vi "Authentication.vi"(2 "password":string, 3 "login":string, 4 "Server Data":string[][](array[string])) -> (0 "Index":i32, 1 "IsValid?":bool)   [LabVIEW 2016]
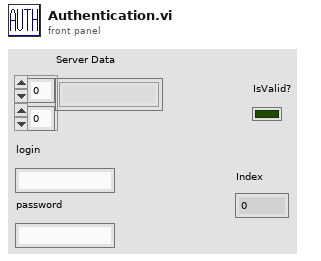
[diagram p1: front panel]
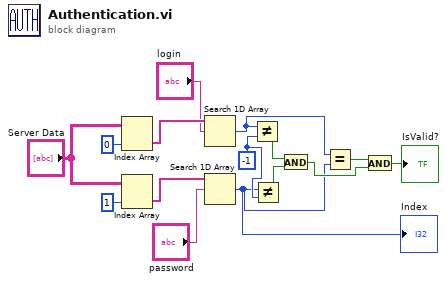
[diagram p0: block diagram]
diagram:
  w8 = -1
  n1 = Index Array(array="Server Data", index (col)=0) -> (element=w12:string[])  [unwired: 1 in]
  n2 = Index Array(array="Server Data", index (col)=1) -> (element=w10:string[])  [unwired: 1 in]
  n3 = Search 1D Array(1D array=w12, element="login") -> (index of element=w5:i32)  [unwired: 1 in]
  n4 = Search 1D Array(1D array=w10, element="password") -> (index of element=w1:i32)  [unwired: 1 in]
  "Index" <- w1
  n5 = Not Equal?(x=w5, y=w8) -> (x != y?=w6:bool)
  n6 = Not Equal?(x=w1, y=w8) -> (x != y?=w7:bool)
  n7 = And(x=w6, y=w7) -> (x .and. y?=w3:bool)
  n8 = Equal?(x=w5, y=w1) -> (x = y?=w4:bool)
  n9 = And(x=w4, y=w3) -> (x .and. y?=→"IsValid?":bool)
